vi "in_2d centered derivatives.vi"(9 "Y column":dbl[](array[numeric]), 10 "X row":dbl[](array[numeric]), 11 "Z matrix":dbl[][](array[numeric])) -> (1 "zderiv12":dbl[][](array[numeric]) format="%_6g", 2 "zderiv2":dbl[][](array[numeric]) format="%_6g", 3 "zderiv1":dbl[][](array[numeric]) format="%_6g")   [LabVIEW 2020, in "NI_Gmath.lvlib"]
uses:
  <vilib>/gmath/NI_Gmath.lvlib
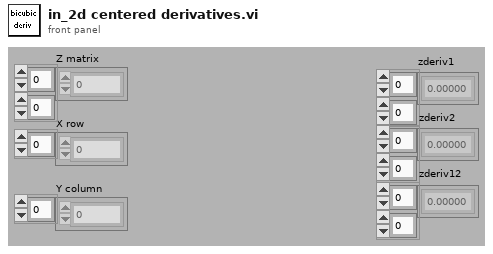
[diagram p1: front panel]
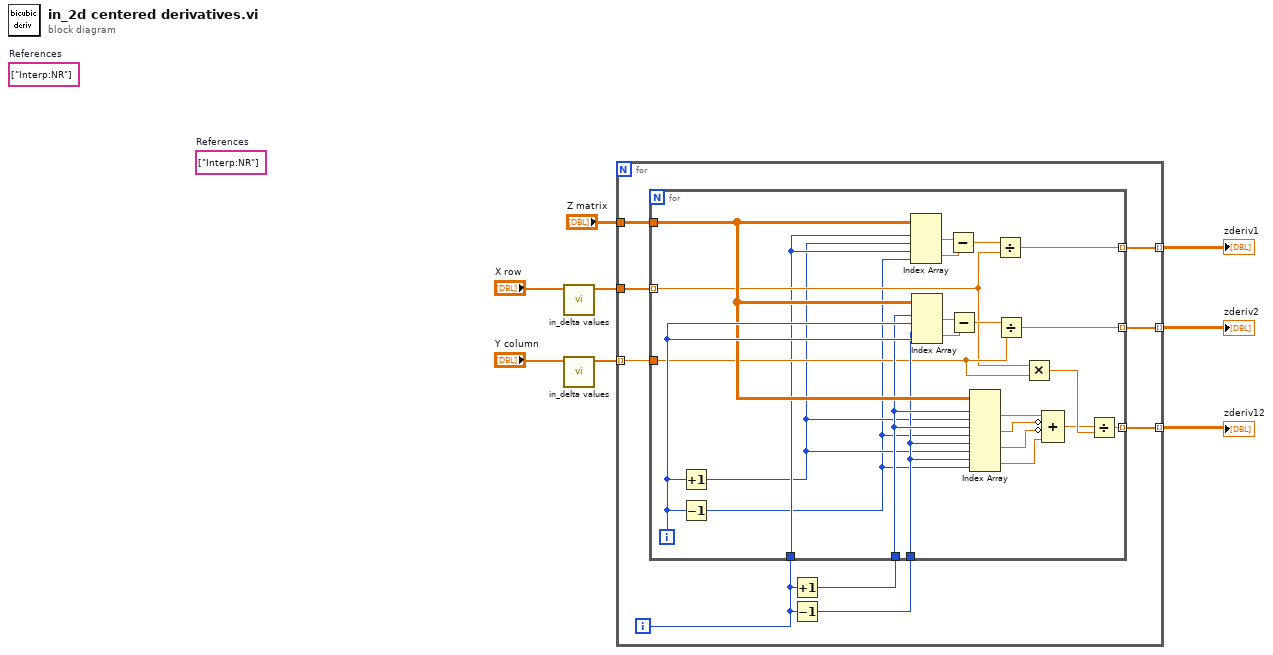
[diagram p0: block diagram]
diagram:
  (unwired) string[] ["Interp:NR"]  # References
  (unwired) string[] ["Interp:NR"]  # References
  n1 = call <vilib>:"in_delta values.vi"("x array"="X row") -> ("x delta values"=w4:dbl[])  [unwired: 10 in]
  n2 = call <vilib>:"in_delta values.vi"("x array"="Y column") -> ("x delta values"=w2:dbl[])  [unwired: 10 in]
  n3 = for {
    tunnel: "Z matrix" -> [w13]
    tunnel: w4 -> [w12]
    tunnel: w2 -> [w17] mode=indexing
    tunnel: [w16] -> w8 mode=indexing
    tunnel: [w15] -> w7 mode=indexing
    tunnel: [w14] -> w6 mode=indexing
    i -> [w11]
    n4 = Increment(x=w11) -> (x+1=w10:i32)
    n5 = Decrement(x=w11) -> (x-1=w9:i32)
    n6 = for {
      tunnel: w13 -> [w34]
      tunnel: w12 -> [w26] mode=indexing
      tunnel: w17 -> [w27]
      tunnel: w11 -> [w22]
      tunnel: [w19] -> w16 mode=indexing
      tunnel: w10 -> [w33]
      tunnel: w9 -> [w32]
      tunnel: [w18] -> w15 mode=indexing
      tunnel: [w23] -> w14 mode=indexing
      i -> [w35]
      n7 = Increment(x=w35) -> (x+1=w21:i32)
      n8 = Decrement(x=w35) -> (x-1=w20:i32)
      n9 = Index Array(array=w34, index (row) #1=w22, index (col) #1=w21, index (row) #2=w22, index (col) #2=w20) -> (element #1=w41:dbl, element #2=w40:dbl)
      n10 = Index Array(array=w34, index (row) #1=w33, index (col) #1=w35, index (row) #2=w32, index (col) #2=w35) -> (element #1=w36:dbl, element #2=w37:dbl)
      n11 = Subtract(x=w41, y=w40) -> (x-y=w39:dbl)
      n12 = Subtract(x=w36, y=w37) -> (x-y=w38:dbl)
      n13 = Index Array(array=w34, index (row) #1=w33, index (col) #1=w21, index (row) #2=w33, index (col) #2=w20, index (row) #3=w32, index (col) #3=w21, index (row) #4=w32, index (col) #4=w20) -> (element #1=w31:dbl, element #2=w30:dbl, element #3=w29:dbl, element #4=w28:dbl)
      n14 = Divide(x=w39, y=w26) -> (x/y=w19:dbl)
      n15 = Divide(x=w38, y=w27) -> (x/y=w18:dbl)
      n16 = Multiply(x=w26, y=w27) -> (x*y=w25:dbl)
      n17 = Compound Arithmetic op=ADD(w31, invert w30, invert w29, w28) -> (w24:dbl)
      n18 = Divide(x=w24, y=w25) -> (x/y=w23:dbl)
    }
  }
  "zderiv1" <- w8
  "zderiv2" <- w7
  "zderiv12" <- w6
